vi "TestExec.Get Fault Code Prefix.vi"(10 "Limit In":T1={"Name"="CodePrefix", "LimType"=enum."None", "LL"="", "UL"="", "Units"="", "FailCode"=0, "FailDesc"=""}) -> (1 "FaultCode Prefix":i32, 2 "Code Prefix Lim Out":T1={"Name"="CodePrefix", "LimType"=enum."None", "LL"="", "UL"="", "Units"="", "FailCode"=0, "FailDesc"=""})   [LabVIEW 2019]
uses:
  Results/Limits/Result.Test Limit Item.ctl
  Results/Result.Limit Type.ctl
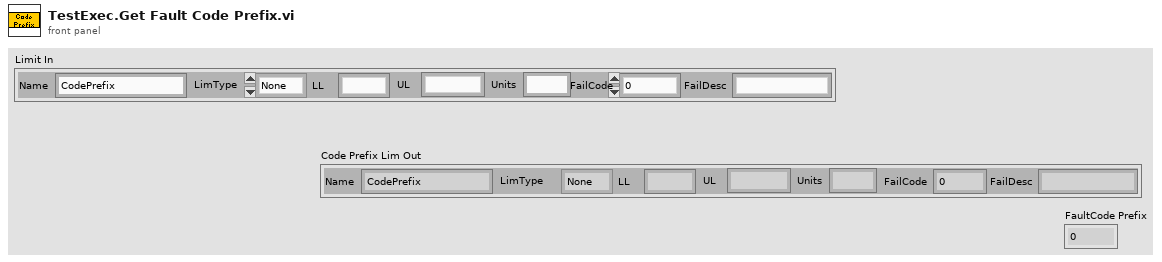
[diagram p1: front panel]
types:
  T1 = typedef "Result.Test Limit Item.ctl" = cluster{"Name":string, "LimType":T2, "LL":string, "UL":string, "Units":string, "FailCode":i32, "FailDesc":string}
  T2 = typedef "Result.Limit Type.ctl" = enum16{"None", "EQ", "NE", "GT", "LT", "GE", "LE", "GTLT", "GELE", "GELT", "GTLE", "LTGT", "LEGE", "LEGT", "LTGE", "Contains", "NotContains"}
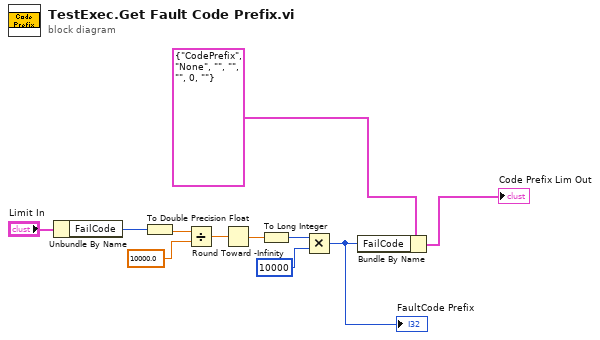
[diagram p0: block diagram]
diagram:
  n1 = Unbundle By Name("Limit In") -> ("FailCode"=w10:i32)
  n2 = To Double Precision Float(number=w10) -> (double precision float=w9:dbl)
  n3 = Divide(x=w9, y=10000.0) -> (x/y=w7:dbl)
  n4 = Round Toward -Infinity(1:w7) -> (0:w6:dbl)
  n5 = To Long Integer(number=w6) -> (32bit integer=w5:i32)
  n6 = Multiply(x=w5, y=10000) -> (x*y=w1:i32)
  "FaultCode Prefix" <- w1
  n7 = Bundle By Name(cluster=T1 {"Name"="CodePrefix", "LimType"=enum."None", "LL"="", "UL"="", "Units"="", "FailCode"=0, "FailDesc"=""} ("Code Prefix Lim Out"), "FailCode"=w1) -> (→"Code Prefix Lim Out":T1)
